vi "LowIF_audiojack.vi"() -> ()   [LabVIEW 2014]
doc: "This example demonstrates how to use the Short-time Fourier Transform (STFT Spectrograms) VI to analyze the Time-Frequency spectrogram."
uses:
  <vilib>/sound2/lvsound2.llb/Sampling Mode.ctl
  <vilib>/Analysis/2dsp.llb/Complex FFT.vi
  <vilib>/sound2/lvsound2.llb/Sound Input Read (DBL).vi
  <vilib>/Analysis/baseanly.llb/Mean (CDB).vi
  <vilib>/Analysis/NI_AALPro.lvlib
  <vilib>/Analysis/NI_AALBase.lvlib
panel:
  in  "scale to beats per min?":bool
  in  "Minimun dB":dbl=-15.0 max=0.0
  in  "dB scale?":bool
  in  "Frequency Range":dbl(slide)=3.2 caption="Beats per Min (x60)" min=1.0 step=0.1 scale=0.0..160.0
  in  "negative frequency?":bool=TRUE
  out "Frequency":dbl[](graph) caption="I/Q Signal"
  in  "bits per sample":i32=16
  in  "number of channels":i32=2
  in  "sample rate (S/s)":dbl=320.0
  in  "data length":i32=6400
  out "I/Q Signal":dynamicdata(graph)
  in  "number of samples/ch":i32=32
  in  "device ID":u32
  in  "Stop":bool
  # "Low-IF interferometry radar data processing"
  # "Version: 2\nZhengyu Peng\nC. Li Lab\nTexas Tech University\nSep. 2015"
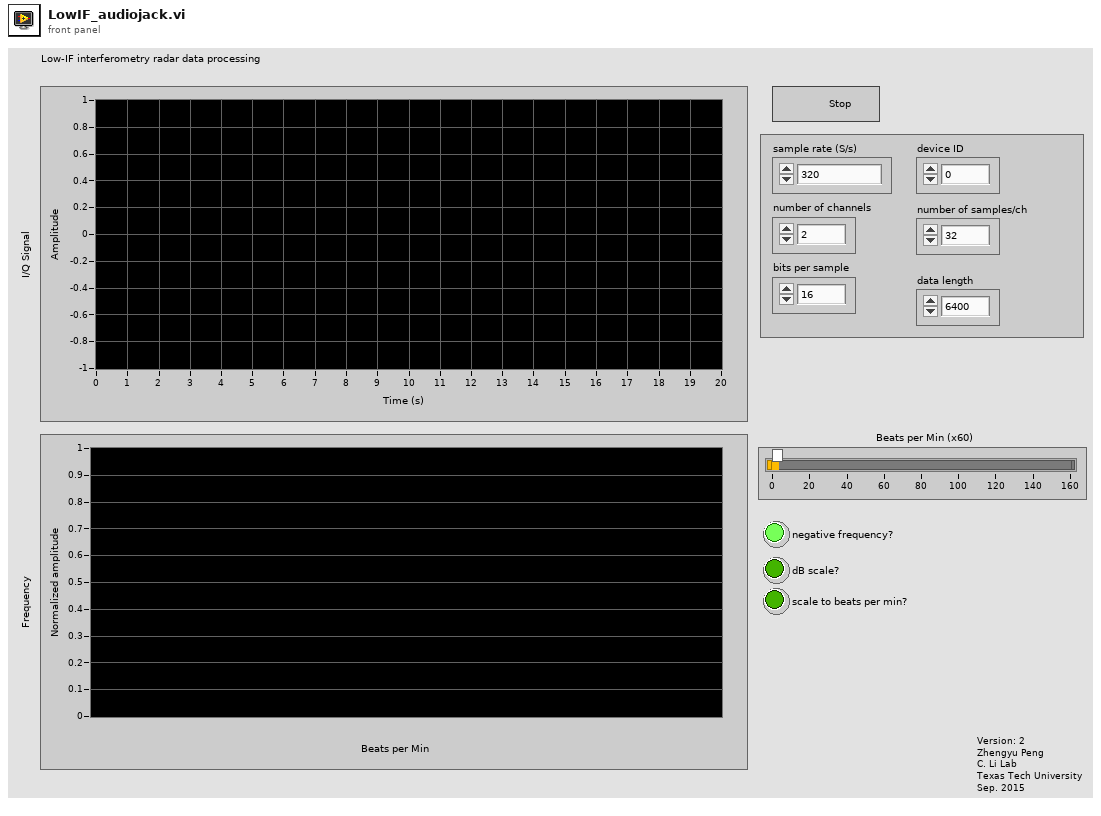
[diagram p1: front panel]
types:
  T1 = typedef "Sampling Mode.ctl" = i32
  T2 = cluster{"sample rate (S/s)":dbl, "number of channels":i32, "bits per sample ":i32}
  T3 = typedef "Sound Input Task ID.ctl" = u32
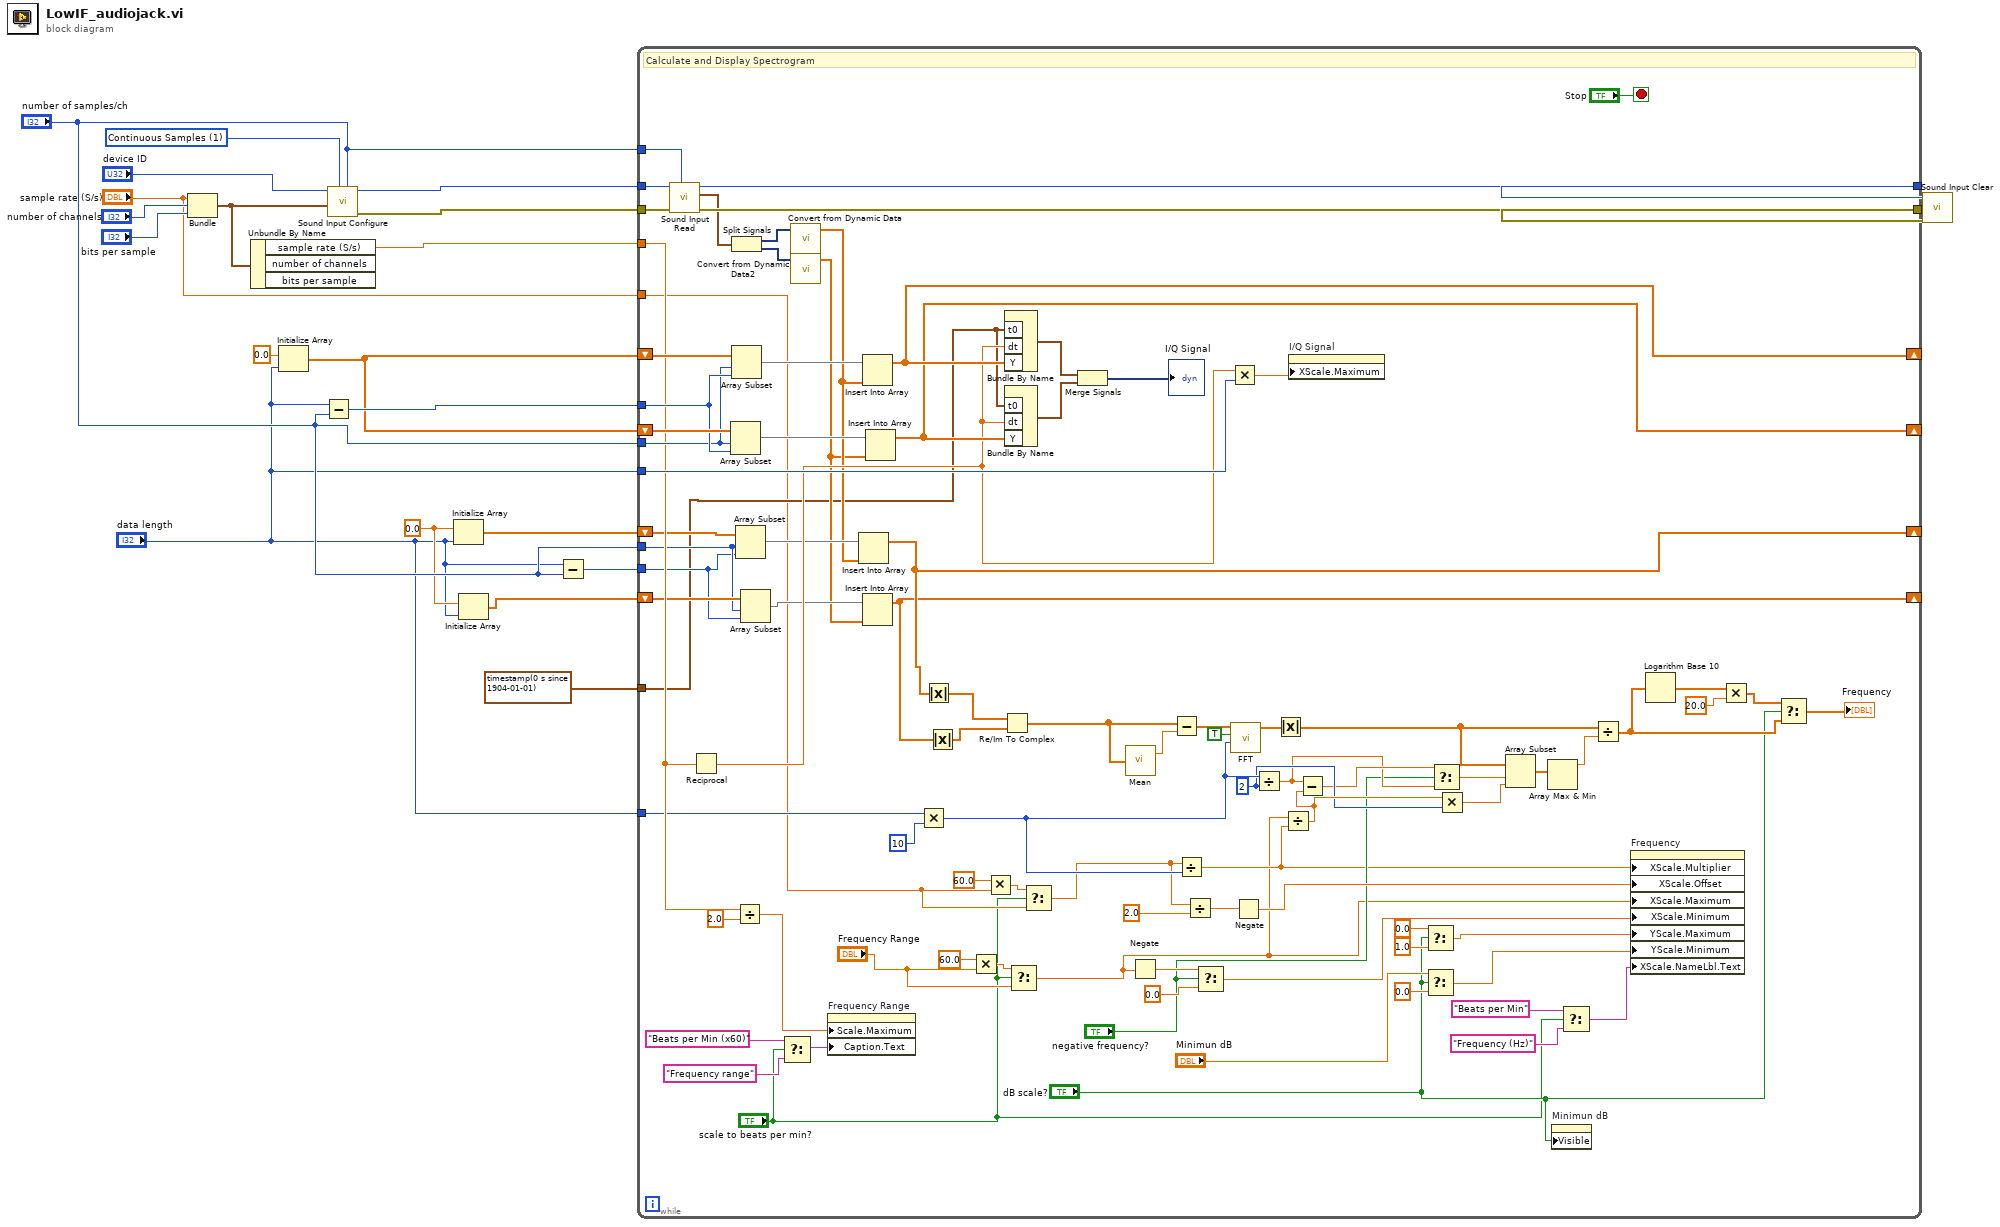
[diagram p0: block diagram]
diagram:
  w3 = T1 1 items=["Finite Samples", "Continuous Samples"] ("sample mode")
  w6 = 0.0 ("element")
  n1 = Bundle("sample rate (S/s)"="sample rate (S/s)", "number of channels"="number of channels", "bits per sample"="bits per sample") -> (w10:T2)  [unwired: 1 in]
  n2 = Unbundle By Name(w10) -> ("sample rate (S/s)"=w13:dbl)  [unwired: 2 out]
  n3 = Initialize Array(0.0 ("element"), "data length") -> (w14:dbl[])
  n4 = Subtract(x="data length", y="number of samples/ch") -> (x-y=w15:i32)
  n5 = call <vilib>:"Sound Input Configure.vi"("number of samples/ch"="number of samples/ch", "sample mode"=w3, "sound format"=w10, "device ID"="device ID") -> ("error out"=w19:errorcluster, "task ID"=w20:T3)  [unwired: 6 in]
  n6 = Initialize Array(w6, "data length") -> (w9:dbl[])
  n7 = Initialize Array(w6, "data length") -> (w5:dbl[])
  n8 = Subtract(x="data length", y="number of samples/ch") -> (x-y=w8:i32)
  n9 = while {
    tunnel: w20 -> [w111]
    tunnel: "number of samples/ch" -> [w110]
    tunnel: w19 -> [w109]
    tunnel: [w108] -> w18
    tunnel: [w107] -> w17
    shift-right: [w91] -> _
    shift-left: w14 -> [w103]
    tunnel: w15 -> [w100]
    shift-right: [w90] -> _
    shift-left: w14 -> [w101]
    tunnel: "number of samples/ch" -> [w97]
    tunnel: w13 -> [w93]
    tunnel: "data length" -> [w95]
    tunnel: "data length" -> [w74]
    tunnel: "sample rate (S/s)" -> [w36]
    shift-right: [w25] -> _
    shift-left: w9 -> [w82]
    tunnel: w8 -> [w77]
    tunnel: "number of samples/ch" -> [w78]
    shift-right: [w23] -> _
    shift-left: w5 -> [w79]
    tunnel: timestamp(0 s since 1904-01-01) ("t0") -> [w71]
    stop <- "Stop" stop-if-true
    w60 = 2 ("y")
    # "Calculate and Display Spectrogram"
    n10 = call-poly <vilib>:"Sound Input Read.vi"("number of samples/ch"=w110, "error in (no error)"=w109, "task ID"=w111) -> ("error out"=w107:errorcluster, "data"=w104:waveform(dbl)[], "task ID out"=w108:T3)  [unwired: 6 in]
    n11 = Reciprocal(x=w93) -> (1/x=w86:dbl)
    n12 = Array Subset(array=w101, index=w97, length=w100) -> (w99:dbl[])
    n13 = Split Signals(w104) -> (w106:dynamicdata, w105:dynamicdata)  [unwired: 2 out]
    n14 = Array Subset(array=w103, index=w97, length=w100) -> (w102:dbl[])
    n15 = Divide(x=w93, y=2.0) -> (x/y=w70:dbl)
    n16 = Array Subset(array=w82, index=w78, length=w77) -> (w81:dbl[])
    n17 = Array Subset(array=w79, index=w78, length=w77) -> (w76:dbl[])
    n18 = Select(t="Beats per Min (x60)" ("X Scale.Name Label.Text"), s="scale to beats per min?", f="Frequency range" ("X Scale.Name Label.Text")) -> (s? t:f=w28:string)
    n19 = call "Convert from Dynamic Data"("Dynamic Data Type"=w106) -> ("Array"=w80:dbl[])  [unwired: 3 out]
    n20 = call "Convert from Dynamic Data2"("Dynamic Data Type"=w105) -> ("Array"=w75:dbl[])  [unwired: 3 out]
    n21 = property on="Frequency Range" class="Slide (strict)"("Scale.Maximum"=w70, "Caption.Text"=w28) -> ()  [unwired: 2 in, 2 out]
    n22 = Insert Into Array(array=w81, new element=w80) -> (w25:dbl[])  [unwired: 1 in]
    n23 = Insert Into Array(array=w102, new element=w80) -> (w91:dbl[])  [unwired: 1 in]
    n24 = Insert Into Array(array=w76, new element=w75) -> (w23:dbl[])  [unwired: 1 in]
    n25 = Insert Into Array(array=w99, new element=w75) -> (w90:dbl[])  [unwired: 1 in]
    n26 = Multiply(x=w74, y=10) -> (x*y=w63:i32)
    n27 = Absolute Value(x=w25) -> (abs(x)=w24:dbl[])
    n28 = Absolute Value(x=w23) -> (abs(x)=w22:dbl[])
    n29 = Multiply(x=60.0, y="Frequency Range") -> (x*y=w34:dbl)
    n30 = Multiply(x=60.0, y=w36) -> (x*y=w39:dbl)
    n31 = Re/Im To Complex(1:w22, 2:w24) -> (0:w26:cdb[])
    n32 = Bundle By Name("t0"=w71, "dt"=w86, "Y"=w91) -> (w98:waveform(dbl))  [unwired: 1 out]
    n33 = Bundle By Name("t0"=w71, "dt"=w86, "Y"=w90) -> (w96:waveform(dbl))  [unwired: 1 out]
    n34 = Select(t=w34, s="scale to beats per min?", f="Frequency Range") -> (s? t:f=w33:dbl)
    n35 = Select(t=w39, s="scale to beats per min?", f=w36) -> (s? t:f=w37:dbl)
    n36 = Merge Signals(w98, w96) -> (→"I/Q Signal":dynamicdata)
    n37 = call-poly <vilib>:"Mean.vi"("X"=w26) -> ("mean"=w89:cdb)  [unwired: 1 out]
    n38 = Negate(x=w33) -> (-x=w67:dbl)
    n39 = Subtract(x=w26, y=w89) -> (x-y=w72:cdb[])
    n40 = Divide(x=w37, y=w63) -> (x/y=w38:dbl)
    n41 = Divide(x=w37, y=2.0) -> (x/y=w84:dbl)
    n42 = Select(t=w67, s="negative frequency?", f=0.0) -> (s? t:f=w69:dbl)
    n43 = Multiply(x=w86, y=w95) -> (x*y=w94:dbl)
    n44 = call-poly <vilib>:"FFT.vi"("FFT size"=w63, "shift?"=TRUE, "X"=w72) -> ("FFT {X}"=w87:cdb[])  [unwired: 7 in, 1 out]
    n45 = Negate(x=w84) -> (-x=w83:dbl)
    n46 = Divide(x=w63, y=w60) -> (x/y=w57:dbl)
    n47 = Absolute Value(x=w87) -> (abs(x)=w66:dbl[])
    n48 = Divide(x=w33, y=w38) -> (x/y=w61:dbl)
    n49 = property on="I/Q Signal" class="WFGraph (strict)"("XScale.Maximum"=w94) -> ()  [unwired: 2 in, 2 out]
    n50 = Subtract(x=w57, y=w61) -> (x-y=w58:dbl)
    n51 = Select(t=0.0, s="dB scale?", f=1.0) -> (s? t:f=w47:dbl)
    n52 = Select(t="Minimun dB", s="dB scale?", f=0.0) -> (s? t:f=w51:dbl)
    n53 = Select(t=w58, s="negative frequency?", f=w57) -> (s? t:f=w59:dbl)
    n54 = Multiply(x=w61, y=w60) -> (x*y=w62:dbl)
    n55 = Array Subset(array=w66, index=w59, length=w62) -> (w65:dbl[])
    n56 = Array Max & Min(array=w65) -> (max value=w64:dbl)  [unwired: 3 out]
    n57 = property on="Minimun dB" class="DigNum (strict)"("Visible"="dB scale?") -> ()  [unwired: 2 in, 2 out]
    n58 = Select(t="Beats per Min" ("X Scale.Name Label.Text"), s="scale to beats per min?", f="Frequency (Hz)" ("X Scale.Name Label.Text")) -> (s? t:f=w42:string)
    n59 = Divide(x=w66, y=w64) -> (x/y=w45:dbl[])
    n60 = property on="Frequency" class="WFGraph (strict)"("XScale.Multiplier"=w38, "XScale.Offset"=w83, "XScale.Maximum"=w33, "XScale.Minimum"=w69, "YScale.Maximum"=w47, "YScale.Minimum"=w51, "XScale.NameLbl.Text"=w42) -> ()  [unwired: 2 in, 2 out]
    n61 = Logarithm Base 10(1:w45) -> (0:w55:dbl[])
    n62 = Multiply(x=w55, y=20.0) -> (x*y=w53:dbl[])
    n63 = Select(t=w53, s="dB scale?", f=w45) -> (s? t:f=→"Frequency":dbl[])
  }
  n64 = call <vilib>:"Sound Input Clear.vi"("error in (no error)"=w17, "task ID"=w18) -> ()  [unwired: 9 in, 1 out]
